vi "Obtain Queue.vi"(8 "error in (no error)":errorcluster, 10 "Sharing Queue":refnum<queue>, 11 "OOQMH in":refnum<class "OOQMH.lvclass">) -> (0 "error out":errorcluster, 3 "OOQMH out":refnum<class "OOQMH.lvclass">)   [LabVIEW 2024, in "OOQMH.lvlib" / "OOQMH.lvclass"]
uses:
  OOQMH.lvclass
  Message/Message.lvclass
  OOQMH.lvclass/OOQMH.ctl
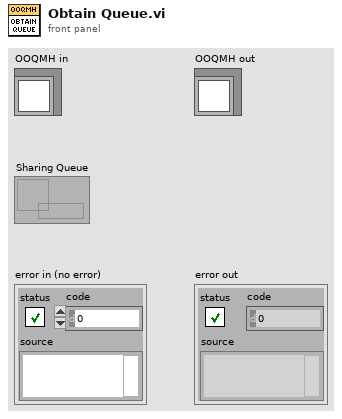
[diagram p1: front panel]
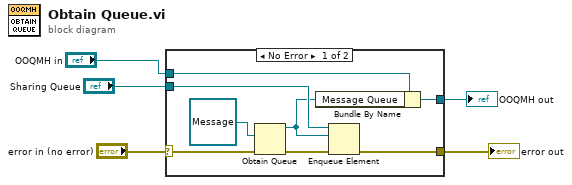
[diagram p0: block diagram]
diagram:
  n1 = case shown="No Error" "error in (no error)" {
    selector: "error in (no error)" -> [w13 w15]
    tunnel: [w8 w15] -> w4
    tunnel: [w10 w14] -> w2
    tunnel: "OOQMH in" -> [w11 w14]
    tunnel: "Sharing Queue" -> [w7 _]
    frame No Error {
      n2 = Obtain Queue(element data type=refnum<class "Message.lvclass"> refnum ("OOQMH.lvlib:Message.lvclass"), error in (no error)=w13) -> (queue out=w6:refnum<queue>, error out=w9:errorcluster)  [unwired: 3 in, 1 out]
      n3 = Bundle By Name(cluster=w11, "Message Queue"=w6) -> (w10:refnum<class "OOQMH.lvclass">)
      n4 = Enqueue Element(queue=w7, element=w6, error in (no error)=w9) -> (error out=w8:errorcluster)  [unwired: 1 in, 2 out]
    }
    frame Error {
    }
  }
  "error out" <- w4
  "OOQMH out" <- w2
